vi "GetOCUCommands.vi"(8 "error in (no error)":errorcluster, 9 "MissionArray":refnum<class "GenericMission.lvclass">[](array[class]), 10 "Mission To Delete":refnum<queue>, 11 "Missions From OCU":refnum<queue>) -> (0 "error out":errorcluster, 2 "First mission changed?":bool, 3 "UpdatedMissionArray":refnum<class "GenericMission.lvclass">[](array[class]))   [LabVIEW 2013]
doc: "Add a mission or delets a misison from the CurrentMissions array when an item to add or delete is put into the respecitve queues\n\nUpdate (3/12/14) :\nThe last mission in the array should always be the default idle mission. \n-KK"
uses:
  Classes/Missions/GenericMission/GenericMission.lvclass
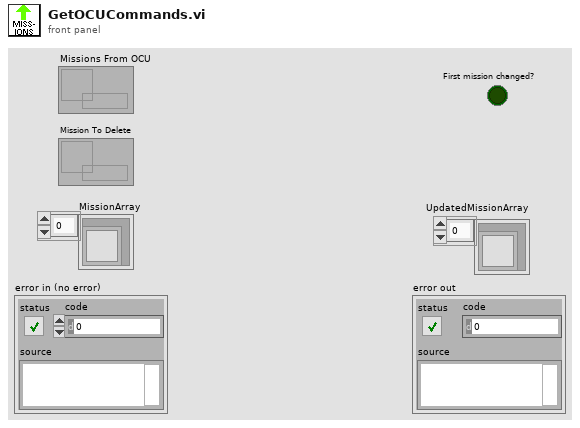
[diagram p1: front panel]
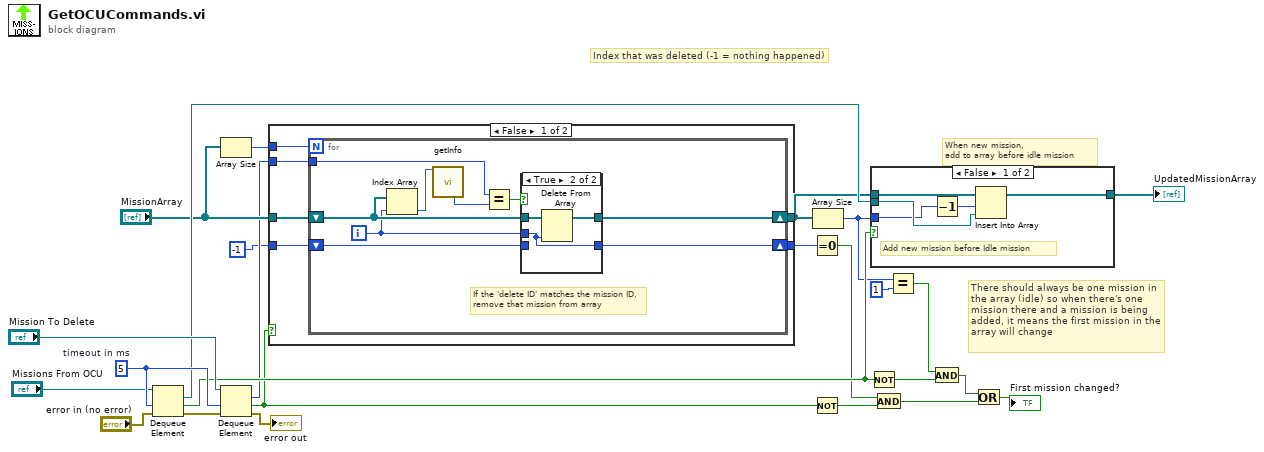
[diagram p0: block diagram]
diagram:
  w24 = 5  # timeout in ms
  # "Index that was deleted (-1 = nothing happened)"
  # "There should always be one mission in the array (idle) so when there's one mission there and a mission is being added, it means the first mission in the array will change"
  # "When new mission,\nadd to array before idle mission"
  n1 = Dequeue Element(queue="Missions From OCU", timeout in ms (-1)=w24, error in (no error)="error in (no error)") -> (element=w22:refnum<class "GenericMission.lvclass">, timed out?=w17:bool, error out=w20:errorcluster)  [unwired: 1 out]
  n2 = Array Size(array="MissionArray") -> (size(s)=w8:i32)
  n3 = Dequeue Element(queue="Mission To Delete", timeout in ms (-1)=w24, error in (no error)=w20) -> (element=w6:i32, timed out?=w1:bool, error out=→"error out":errorcluster)  [unwired: 1 out]
  n4 = case shown="False" w1 {
    tunnel: [w31 w46] -> w9
    tunnel: w8 -> [w30 _]
    tunnel: "MissionArray" -> [w29 w46]
    tunnel: w6 -> [w28 _]
    tunnel: [w27 w47] -> w5
    tunnel: -1 -> [w26 w47]
    frame False {
      n5 = for {
        N: w30 -> [_]
        shift-right: [w36] -> w31
        shift-left: w29 -> [w38]
        tunnel: w28 -> [w32]
        shift-right: [w34] -> w27
        shift-left: w26 -> [w35]
        i -> [w37]
        # "If the 'delete ID' matches the mission ID, remove that mission from array"
        n6 = Index Array(array=w38, index=w37) -> (element=w40:refnum<class "GenericMission.lvclass">)
        n7 = call-dynamic "getInfo.vi"("GenericMission in"=w40) -> ("ID#"=w33:i16)  [unwired: 6 in, 8 out]
        n8 = Equal?(x=w32, y=w33) -> (x = y?=w39:bool)
        n9 = case shown="True" w39 {
          tunnel: w38 -> [w42 w45]
          tunnel: w37 -> [_ w43]
          tunnel: [w42 w44] -> w36
          tunnel: w35 -> [w41 _]
          tunnel: [w41 w43] -> w34
          frame False {
          }
          frame True {
            n10 = Delete From Array(array=w45, index=w43) -> (array with subset deleted=w44:refnum<class "GenericMission.lvclass">[])  [unwired: 1 in, 1 out]
          }
        }
      }
    }
    frame True {
      # "If the queue call timed out, there are no missions to delete, so don't delete anything"
    }
  }
  n11 = Equal To 0?(x=w5) -> (x = 0?=w3:bool)
  n12 = Not(x=w1) -> (.not. x?=w4:bool)
  n13 = Array Size(array=w9) -> (size(s)=w14:i32)
  n14 = Not(x=w17) -> (.not. x?=w16:bool)
  n15 = case shown="False" w17 {
    tunnel: w22 -> [w52 _]
    tunnel: w9 -> [w50 w53]
    tunnel: [w51 w53] -> w18
    tunnel: w14 -> [w48 _]
    frame False {
      # "Add new mission before Idle mission"
      n16 = Decrement(x=w48) -> (x-1=w49:i32)
      n17 = Insert Into Array(array=w50, index=w49, new element=w52) -> (w51:refnum<class "GenericMission.lvclass">[])
    }
    frame True {
    }
  }
  "UpdatedMissionArray" <- w18
  n18 = And(x=w3, y=w4) -> (x .and. y?=w11:bool)
  n19 = Equal?(x=w14, y=1) -> (x = y?=w15:bool)
  n20 = And(x=w15, y=w16) -> (x .and. y?=w12:bool)
  n21 = Or(x=w12, y=w11) -> (x .or. y?=→"First mission changed?":bool)
